vi "Generate general triggers.vi"(7 "Experiment start":bool, 9 "Inter-loop signals":T2, 10 "General trig. pulse width":T4={"Trigger 1 function"=enum."Encoder trigger", "Pulse width (ticks)-Line Trig."=0, "Pulse width (ticks)-Frame/Cycle Trig."=0, "Pulse width (ticks)-Trial trig."=0, "Pulse width (ticks)-Start of Exp. trig."=80000}, 11 "FPGA state":T3) -> (1 "Trigger lines value":T1, 3 "Unmodified signal values":T1)   [LabVIEW 2020]
uses:
  FPGA Typedefs/General trig pulse width.ctl
  Typedefs/Trigger 1 selector enum.ctl
  FPGA Typedefs/Image State.ctl
  FPGA Typedefs/PXI Trigger lines value cluster.ctl
  FPGA Typedefs/Inter-loop signals.ctl
panel:
  # "(80=1us)"
  # "(80=1us)"
  # "(80000=1ms)"
  # "(80000=1ms)"
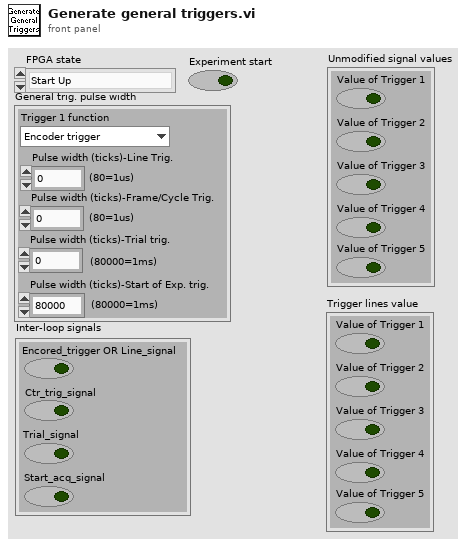
[diagram p1: front panel]
types:
  T1 = typedef "PXI Trigger lines value cluster.ctl" = cluster{"Value of Trigger 1":bool, "Value of Trigger 2":bool, "Value of Trigger 3":bool, "Value of Trigger 4":bool, "Value of Trigger 5":bool}
  T2 = typedef "Inter-loop signals.ctl" = cluster{"Encored_trigger OR Line_signal":bool, "Ctr_trig_signal":bool, "Trial_signal":bool, "Start_acq_signal":bool}
  T3 = typedef "Image State.ctl" = enum16{"Start Up", "Wait for Trigger", "Wait N after Trigger", "DAQ Pointing", "DAQ Scan", "Reference Scan", "Pointing AOL Fill", "Scan AOL FILL", "Reference AOL Fill"}
  T4 = typedef "General trig pulse width.ctl" = cluster{"Trigger 1 function":T5, "Pulse width (ticks)-Line Trig.":u32, "Pulse width (ticks)-Frame/Cycle Trig.":u32, "Pulse width (ticks)-Trial trig.":u32, "Pulse width (ticks)-Start of Exp. trig.":u32}
  T5 = typedef "Trigger 1 selector enum.ctl" = enum16{"Encoder trigger", "Line trigger", "Control system's ref frame acknowledgement"}
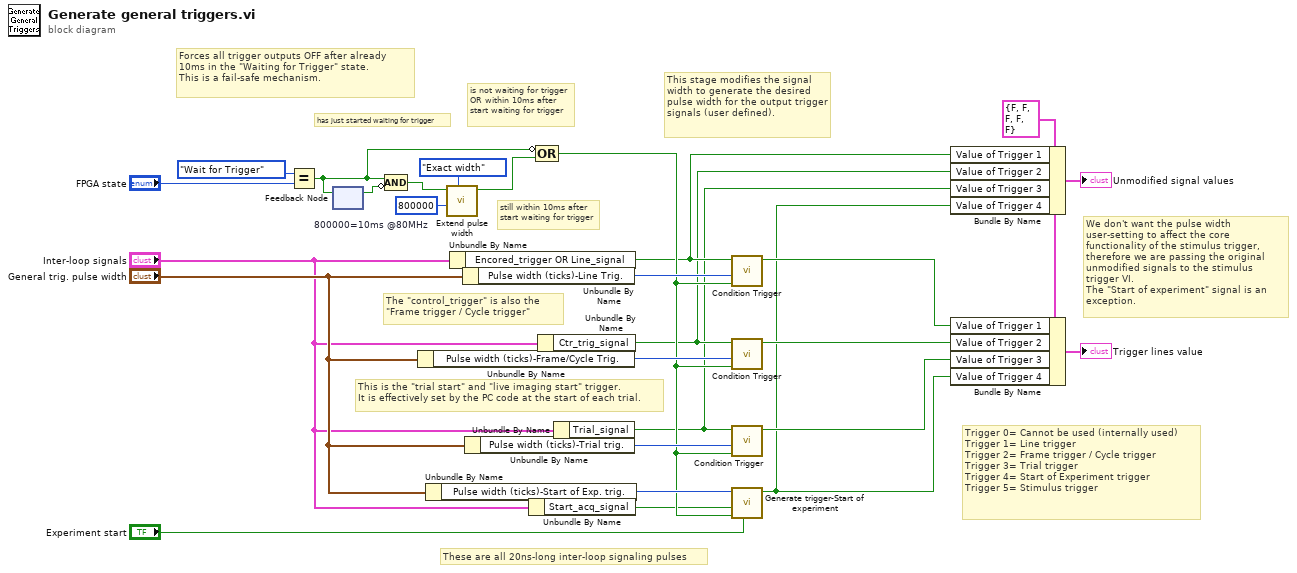
[diagram p0: block diagram]
diagram:
  w7 = u32 800000  # 800000=10ms @80MHz
  w8 = T1 {"Value of Trigger 1"=FALSE, "Value of Trigger 2"=FALSE, "Value of Trigger 3"=FALSE, "Value of Trigger 4"=FALSE, "Value of Trigger 5"=FALSE}
  # "still within 10ms after start waiting for trigger"
  # "has just started waiting for trigger"
  # "is not waiting for trigger OR within 10ms after start waiting for trigger"
  # "Forces all trigger outputs OFF after already 10ms in the \"Waiting for Trigger\" state.\nThis is a fail-safe mechanism."
  # "Trigger 0= Cannot be used (internally used)\nTrigger 1= Line trigger\nTrigger 2= Frame trigger / Cycle trigger\nTrigger 3= Trial trigger\nTrigger 4= Start of Experiment trigger\nTrigger 5= Stimulus trigger"
  # "This stage modifies the signal width to generate the desired pulse width for the output trigger signals (user defined)."
  # "We don't want the pulse width user-setting to affect the core functionality of the stimulus trigger, therefore we are passing the original unmodified signals to the stimulus trigger VI.\nThe \"Start of experiment\" signal is an exception."
  # "These are all 20ns-long inter-loop signaling pulses"
  # "The \"control_trigger\" is also the \"Frame trigger / Cycle trigger\""
  # "This is the \"trial start\" and \"live imaging start\" trigger.\nIt is effectively set by the PC code at the start of each trial."
  n1 = Equal?(x=Image_State."Wait for Trigger", y="FPGA state") -> (x = y?=w1:bool)
  n2 = feedback #1() -> (w4:bool)  [unwired: 1 in]
  n3 = feedback-in #1(w1) -> ()
  n4 = Compound Arithmetic op=AND(w1, invert w4) -> (w3:bool)
  n5 = Unbundle By Name("General trig. pulse width") -> ("Pulse width (ticks)-Frame/Cycle Trig."=w24:u32)
  n6 = Unbundle By Name("General trig. pulse width") -> ("Pulse width (ticks)-Start of Exp. trig."=w27:u32)
  n7 = call "Extend pulse width.vi"("Function"=enum16{"Minimum width", "Exact width"}."Exact width", "Pulse width (ticks)(80000=1ms @80MHz)"=w7, "Input signal"=w3) -> ("Output signal"=w2:bool)  [unwired: 8 in]
  n8 = Unbundle By Name("Inter-loop signals") -> ("Encored_trigger OR Line_signal"=w13:bool)
  n9 = Unbundle By Name("General trig. pulse width") -> ("Pulse width (ticks)-Line Trig."=w23:u32)
  n10 = Unbundle By Name("General trig. pulse width") -> ("Pulse width (ticks)-Trial trig."=w25:u32)
  n11 = Unbundle By Name("Inter-loop signals") -> ("Start_acq_signal"=w16:bool)
  n12 = Compound Arithmetic op=OR(invert w1, w2) -> (w18:bool)
  n13 = Unbundle By Name("Inter-loop signals") -> ("Ctr_trig_signal"=w12:bool)
  n14 = Unbundle By Name("Inter-loop signals") -> ("Trial_signal"=w11:bool)
  n15 = call "Condition Trigger.vi"("Acquiring"=w18, "Pulse width (ticks)-Trial trig."=w23, "Input signal"=w13) -> ("Output signal"=w19:bool)  [unwired: 8 in]
  n16 = call "Condition Trigger.vi"("Acquiring"=w18, "Pulse width (ticks)-Trial trig."=w24, "Input signal"=w12) -> ("Output signal"=w17:bool)  [unwired: 8 in]
  n17 = call "Condition Trigger.vi"("Acquiring"=w18, "Pulse width (ticks)-Trial trig."=w25, "Input signal"=w11) -> ("Output signal"=w10:bool)  [unwired: 8 in]
  n18 = call "Generate trigger-Start of experiment.vi"("Experiment start"="Experiment start", "Acquiring"=w18, "start_ac_pulse"=w16, "Pulse width (ticks) -\"Start of Acq\" Trigger"=w27) -> ("\"Start of Acquisition\" trigger"=w9:bool)  [unwired: 7 in]
  n19 = Bundle By Name(cluster=w8, "Value of Trigger 1"=w13, "Value of Trigger 2"=w12, "Value of Trigger 3"=w11, "Value of Trigger 4"=w9) -> (→"Unmodified signal values":T1)
  n20 = Bundle By Name(cluster=w8, "Value of Trigger 1"=w19, "Value of Trigger 2"=w17, "Value of Trigger 3"=w10, "Value of Trigger 4"=w9) -> (→"Trigger lines value":T1)
